vi "IPS120_act.vi"(2 "Action":u16, 3 "Set Rate":dbl, 4 "Set Point":dbl, 5 "Address":T1) -> (0 "Target B":string, 1 "Rate":string)   [LabVIEW 2012]
uses:
  Oxford_itc503/BUSGEN.LLB/OxfordAddress.ctl
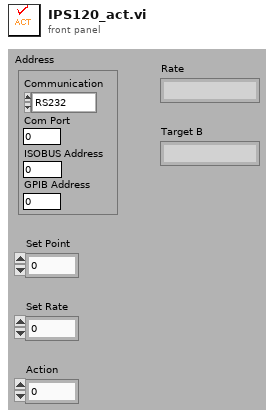
[diagram p1: front panel]
types:
  T1 = typedef "OxfordAddress.ctl" = cluster{"Com Port":i32, "ISOBUS Address":i32, "GPIB Address":i16, "Communication":enum16{"RS232", "ISOBUS", "GPIB", "Gateway"}}
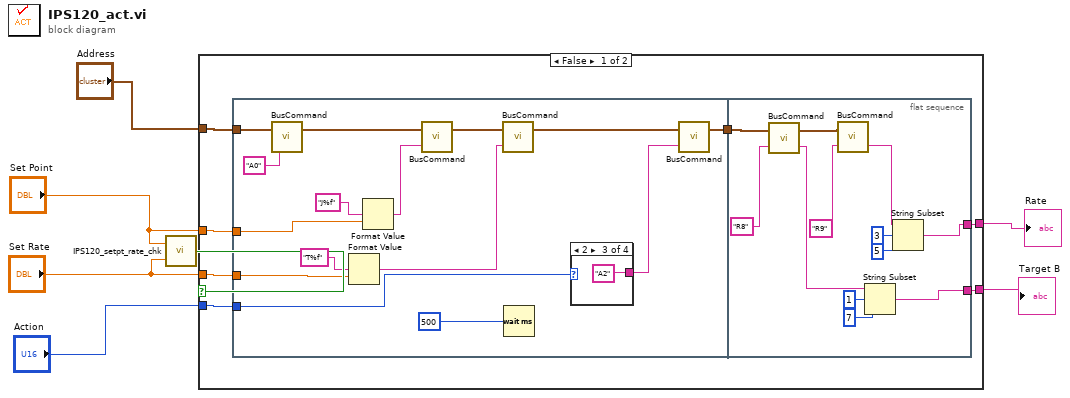
[diagram p0: block diagram]
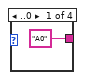
[diagram p2: hidden frame]
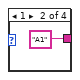
[diagram p3: hidden frame]
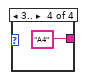
[diagram p4: hidden frame]
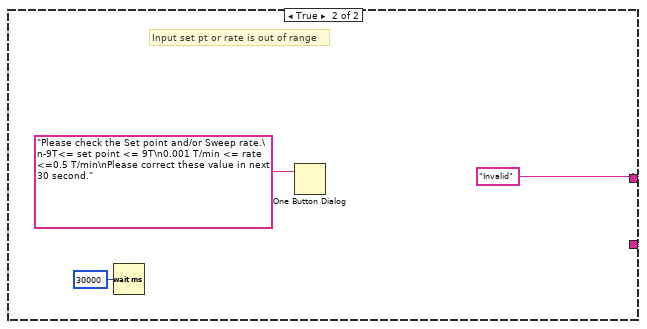
[diagram p5: hidden frame]
diagram:
  n1 = call "IPS120_setpt_rate_chk.vi"("Set Rate"="Set Rate", "Set Point"="Set Point") -> ("chk set pt and rate"=w5:bool)
  n2 = case shown="False" w5 {
    tunnel: "Action" -> [w11 _]
    tunnel: "Set Point" -> [w14 _]
    tunnel: "Set Rate" -> [w13 _]
    tunnel: "Address" -> [w12 _]
    tunnel: [w10 w46] -> w6
    tunnel: [w9 w46] -> w7
    frame False {
      n3 = flat-sequence {
        tunnel: w14 -> [w18]
        tunnel: w13 -> [w17]
        tunnel: w12 -> [w19]
        tunnel: w11 -> [w21]
        tunnel: [w15] -> w8
        tunnel: [w36] -> w9
        tunnel: [w35] -> w10
        tunnel: w8 -> [w34]
        frame #0 {
          n4 = call "BusCommand.vi"("Command"="A0", "Instrument address (in)"=w19) -> ("Instrument address (out)"=w16:T1)  [unwired: 1 out]
          n5 = Format Value(format string="T%f", value (0)=w17) -> (output string=w23:string)  [unwired: 1 in]
          n6 = Format Value(format string="J%f", value (0)=w18) -> (output string=w25:string)  [unwired: 1 in]
          n7 = call "BusCommand.vi"("Command"=w25, "Instrument address (in)"=w16) -> ("Instrument address (out)"=w24:T1)  [unwired: 1 out]
          n8 = call "BusCommand.vi"("Command"=w23, "Instrument address (in)"=w24) -> ("Instrument address (out)"=w22:T1)  [unwired: 1 out]
          n9 = Wait (ms)(milliseconds to wait=u32 500) -> ()  [unwired: 1 out]
          n10 = case shown="2" w21 {
            tunnel: ["A0" "A1" "A2" "A4"] -> w20
            frame ..0 {
            }
            frame 1 {
            }
            frame 2 {
            }
            frame 3.. {
            }
          }
          n11 = call "BusCommand.vi"("Command"=w20, "Instrument address (in)"=w22) -> ("Instrument address (out)"=w15:T1)  [unwired: 1 out]
        }
        frame #1 {
          n12 = call "BusCommand.vi"("Command"="R8", "Instrument address (in)"=w34) -> ("Reply"=w40:string, "Instrument address (out)"=w43:T1)
          n13 = call "BusCommand.vi"("Command"="R9", "Instrument address (in)"=w43) -> ("Reply"=w39:string)  [unwired: 1 out]
          n14 = String Subset(string=w40, offset (0)=1, length (rest)=7 ("length (rest)")) -> (substring=w35:string)
          n15 = String Subset(string=w39, offset (0)=3, length (rest)=5 ("length (rest)")) -> (substring=w36:string)
        }
      }
    }
    frame True {
      w46 = "Invalid" ("Reply")
      # "Input set pt or rate is out of range"
      n16 = Wait (ms)(milliseconds to wait=u32 30000) -> ()  [unwired: 1 out]
      n17 = One Button Dialog(message="Please check the Set point and/or Sweep rate.\n-9T<= set point <= 9T\n0.001 T/min <= rate <=0.5 T/min\nPlease correct these value in next 30 second.") -> ()  [unwired: 1 in, 1 out]
    }
  }
  "Rate" <- w7
  "Target B" <- w6
